vi "Standard Event Register Query.vi"(0 "VISA resource name":refnum<visa-resource-name>, 11 "error in (no error)":errorcluster) -> (4 "VISA resource name out":refnum<visa-resource-name>, 6 "Event Status Register":T1, 15 "error out":errorcluster)   [LabVIEW 2020, in "NH Research Regenerative Test Series.lvlib"]
doc: "Queries the Event Status Register and returns the byte data available in it.\nEach bit represent the occurrence of an event.\n\nEx : Bit 0 is set High when \"Operation Complete\"\n\nBit 0: Operation Complete\nBit 1: Request Control\nBit 2: Query Error\nBit 3: Device Error\nBit 4: Execution Error\nBit 5: Command Error\nBit 6: User Request\nBit 7: Power On"
uses:
  NH Research Regenerative Test Series.lvlib
panel:
  # "Bit 0: Operation Complete\nBit 1: Request Control\nBit 2: Query Error\nBit 3: Device Dependant Error\nBit 4: Execution Error\nBit 5: Command Error\nBit 6: User Request\nBit 7: Power On"
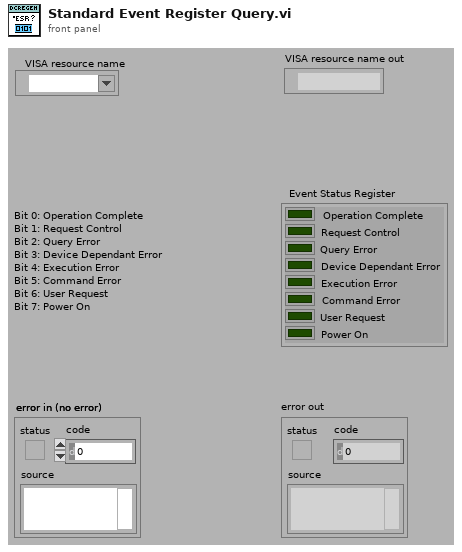
[diagram p1: front panel]
types:
  T1 = cluster{"Operation Complete":bool, "Request Control":bool, "Query Error":bool, "Device Dependant Error":bool, "Execution Error":bool, "Command Error":bool, "User Request":bool, "Power On":bool}
  T2 = cluster{"Boolean array[0]":bool, "Boolean array[1]":bool, "Boolean array[2]":bool, "Boolean array[3]":bool, "Boolean array[4]":bool, "Boolean array[5]":bool, "Boolean array[6]":bool, "Boolean array[7]":bool}
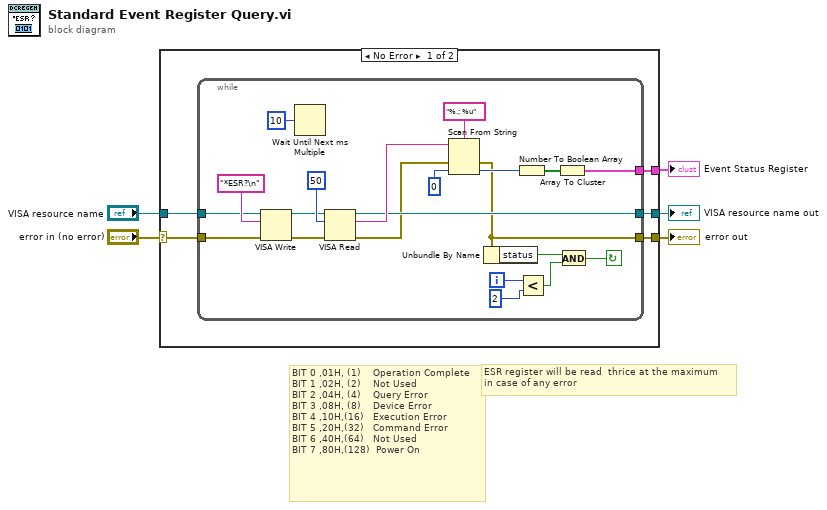
[diagram p0: block diagram]
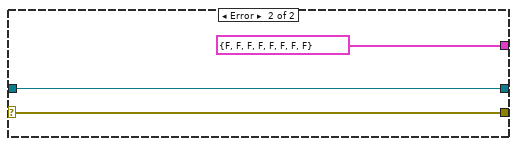
[diagram p2: hidden frame]
diagram:
  # "ESR register will be read  thrice at the maximum\nin case of any error"
  # "BIT 0 ,01H, (1)    Operation Complete\nBIT 1 ,02H, (2)    Not Used\nBIT 2 ,04H, (4)    Query Error\nBIT 3 ,08H, (8)    Device Error\nBIT 4 ,10H,(16)   Execution Error\nBIT 5 ,20H,(32)   Command Error\nBIT 6 ,40H,(64)   Not Used\nBIT 7 ,80H,(128)  Power On"
  n1 = case shown="No Error" "error in (no error)" {
    selector: "error in (no error)" -> [w7 w34]
    tunnel: [w10 T2 {"Boolean array[0]"=FALSE, "Boolean array[1]"=FALSE, "Boolean array[2]"=FALSE, "Boolean array[3]"=FALSE, "Boolean array[4]"=FALSE, "Boolean array[5]"=FALSE, "Boolean array[6]"=FALSE, "Boolean array[7]"=FALSE} ("Boolean array")] -> w1
    tunnel: [w8 w34] -> w2
    tunnel: "VISA resource name" -> [w6 w33]
    tunnel: [w9 w33] -> w4
    frame No Error {
      n2 = while {
        tunnel: [w28] -> w10
        tunnel: w6 -> [w13]
        tunnel: [w27] -> w9
        tunnel: w7 -> [w15]
        tunnel: [w20] -> w8
        i -> [w22]
        stop <- w17 continue-if-true
        n3 = VISA Write(VISA resource name=w13, write buffer="*ESR?\n" ("Command to Send (empty)"), error in (no error)=w15) -> (VISA resource name out=w12:refnum<visa-resource-name>, error out=w14:errorcluster)  [unwired: 1 out]
        n4 = Wait Until Next ms Multiple(millisecond multiple=u32 10) -> ()  [unwired: 1 out]
        n5 = VISA Read(VISA resource name=w12, byte count=u32 50, error in (no error)=w14) -> (VISA resource name out=w27:refnum<visa-resource-name>, read buffer=w30:string, error out=w23:errorcluster)  [unwired: 1 out]
        n6 = Scan From String(format string="%.; %u" ("Format String"), input string=w30, error in=w23, default 1=u8 0 ("default value 1")) -> (error out=w20:errorcluster, output 1=w24:u8)  [unwired: 1 in, 2 out]
        n7 = Unbundle By Name(w20) -> ("status"=w18:bool)
        n8 = Number To Boolean Array(number=w24) -> (Boolean array=w29:bool[])
        n9 = Less?(x=w22, y=2) -> (x < y?=w19:bool)
        n10 = Array To Cluster(array=w29) -> (cluster=w28:T2)
        n11 = And(x=w18, y=w19) -> (x .and. y?=w17:bool)
      }
    }
    frame Error {
    }
  }
  "Event Status Register" <- w1
  "VISA resource name out" <- w4
  "error out" <- w2
